vi "Read Excluded Devices.vi"() -> (0 "error out":errorcluster, 3 "Excluded Devices":string[](array[string]))   [LabVIEW 2020]
uses:
  <vilib>/Utility/sysdir.llb/System Directory Type.ctl
  <vilib>/Utility/config.llb/Read Key (Boolean).vi
  <vilib>/Utility/config.llb/NI_LVConfig.lvlib
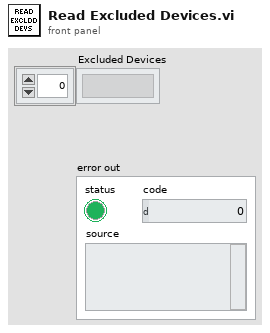
[diagram p1: front panel]
types:
  T1 = typedef "System Directory Type.ctl" = i32
  T2 = typedef "NI_LVConfig.lvlib/Config Data RefNum.ctl" = refnum<k1>
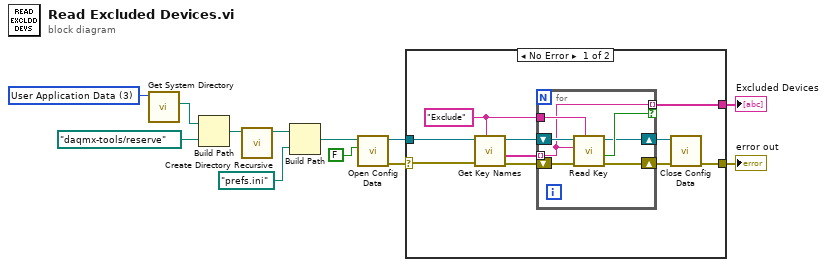
[diagram p0: block diagram]
diagram:
  w12 = T1 3 items=["User Home"=0, "User Desktop"=1, "User Documents"=2, "User Application Data"=3, "User Preferences"=4, "User Temporary"=5, "Public Documents"=6, "Public Application Data"=7, "Public Preferences"=8, "Public Cache"=13, "System Core Libraries"=9, "System Installed Libraries"=10, "Application Files"=11, "Boot Volume Root"=12] ("system directory type")
  n1 = call <vilib>:"Get System Directory.vi"("system directory type"=w12) -> ("system directory"=w11:path)  [unwired: 10 in]
  n2 = Build Path(base path=w11, name or relative path=path "daqmx-tools/reserve") -> (appended path=w9:path)
  n3 = call <vilib>:"Create Directory Recursive.vi"("directory"=w9) -> ("directory copy"=w8:path)  [unwired: 4 in, 2 out]
  n4 = Build Path(base path=w8, name or relative path=path "prefs.ini") -> (appended path=w6:path)
  n5 = call <vilib>:"Open Config Data.vi"("create file if necessary (T)"=FALSE, "configuration file path"=w6) -> ("error out"=w4:errorcluster, "refnum"=w3:T2)  [unwired: 7 in, 1 out]
  n6 = case shown="No Error" w4 {
    selector: w4 -> [w21 w30]
    tunnel: w3 -> [w22 _]
    tunnel: [w14 w30] -> w2
    tunnel: [w13 _] -> w1
    frame No Error {
      w18 = "Exclude" ("section")
      n7 = call <vilib>:"Get Key Names.vi"("section"=w18, "error in (no error)"=w21, "refnum"=w22) -> ("error out"=w19:errorcluster, "key names"=w17:string[], "refnum out"=w20:T2)  [unwired: 5 in, 1 out]
      n8 = for {
        tunnel: w18 -> [w27]
        tunnel: w17 -> [w26] mode=indexing
        tunnel: [w26] -> w13 mode=indexing if=w25
        shift-right: [w24] -> w16
        shift-left: w20 -> [w29]
        shift-right: [w23] -> w15
        shift-left: w19 -> [w28]
        n9 = call-poly <vilib>:"Read Key.vi"("section"=w27, "error in (no error)"=w28, "key"=w26, "refnum"=w29) -> ("error out"=w23:errorcluster, "value"=w25:bool, "refnum out"=w24:T2)  [unwired: 4 in, 1 out]
      }
      n10 = call <vilib>:"Close Config Data.vi"("error in (no error)"=w15, "refnum"=w16) -> ("error out"=w14:errorcluster)  [unwired: 8 in, 1 out]
    }
    frame Error {
    }
  }
  "error out" <- w2
  "Excluded Devices" <- w1
